vi "Main.vi"(8 "error in (no error)":errorcluster, 11 "TomoBase in":refnum<class "Tomo.lvclass">) -> (0 "error out":errorcluster, 3 "component":refnum<class "Tomo.lvclass">)   [LabVIEW 2012, in "Tomo.lvclass"]
doc: "Main VI of the component."
uses:
  Tomo.lvclass
  <vilib>/Distrio/Murmex/Murmex/command_enum.ctl
  Tomo.lvclass/Tomo.ctl
  <vilib>/Distrio/Murmex/InitialiseMessage/InitialiseMessage.lvclass
  <vilib>/Distrio/Murmex/TerminateMessage/TerminateMessage.lvclass
  <vilib>/Distrio/Murmex/ConfigureMessage/ConfigureMessage.lvclass
  <vilib>/Distrio/Murmex/Murmex/update_cluster.ctl
  <vilib>/Distrio/Murmex/StopMessage/StopMessage.lvclass
  <vilib>/Distrio/Murmex/GenericMessage/GenericMessage.lvclass
  <vilib>/Distrio/Murmex/Murmex/Set configure at initialise.vi
  <vilib>/Distrio/Murmex/Murmex/Set log reference.vi
  <vilib>/Distrio/Murmex/Murmex/Set VI reference.vi
  <vilib>/Distrio/Murmex/Message/Add or replace parameter.vi
  <vilib>/Distrio/Murmex/Murmex/Murmex.lvclass
  <vilib>/Distrio/Murmex/Message/Message.lvclass
panel:
  in  "Tab Control":T1(tab)
  out "TB":dbl format="%#_2g"
  out "Tomography progress":dbl(slide) scale=0.0..1.0
  in  "experiment name":string
  in  "Volume map":T2(ring)
  in  "Z step size":dbl[unit]=1e-06
  in  "X step size":dbl[unit]=0.0005
  in  "Y step size":dbl[unit]=0.0005
  in  "number of views":dbl=1.0
  in  "starting angle":dbl[unit]
  in  "button::start":bool
  out "Estimated remaining time":dbl format="- %<%H:%M:%S>t"
  in  "X min":dbl[unit]
  in  "X max":dbl[unit]
  in  "Y min":dbl[unit]
  in  "Y max":dbl[unit]
  in  "Z min":dbl[unit]
  in  "Z max":dbl[unit]
  in  "Custom volume path":path
  in  "generic command":string
  in  "button::send command":bool
  out "log":string
  in  "ID":string="tomo"
  in  "command":T3
  in  "recipient":string
  in  "button::configure":bool
  in  "button::quit":bool
  in  "terminate?":bool
  # "Tomo\n\nImplemented by:\nLudovico Silvestri\nUniversity of Florence, Italy"
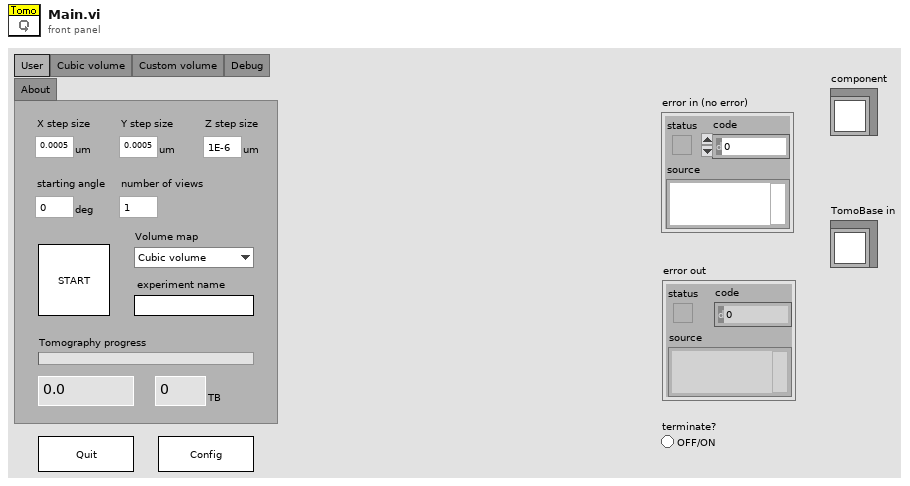
[diagram p1: front panel]
types:
  T1 = enum32{"User", "Cubic volume", "Custom volume", "Debug", "About"}
  T2 = enum16{"Cubic volume", "Custom volume", "Self-generate volume"}
  T3 = typedef "Murmex.lvlib/Murmex.lvclass/command_enum.ctl" = enum16{"null", "initialise", "reset", "terminate", "acknowledge", "update", "inspect", "inform", "proceed", "start", "stop", "fetch", "configure", "generic"}
  T4 = typedef "Murmex.lvlib/Murmex.lvclass/update_cluster.ctl" = cluster{"target ID":string, "key chains":string[], "values":variant[]}
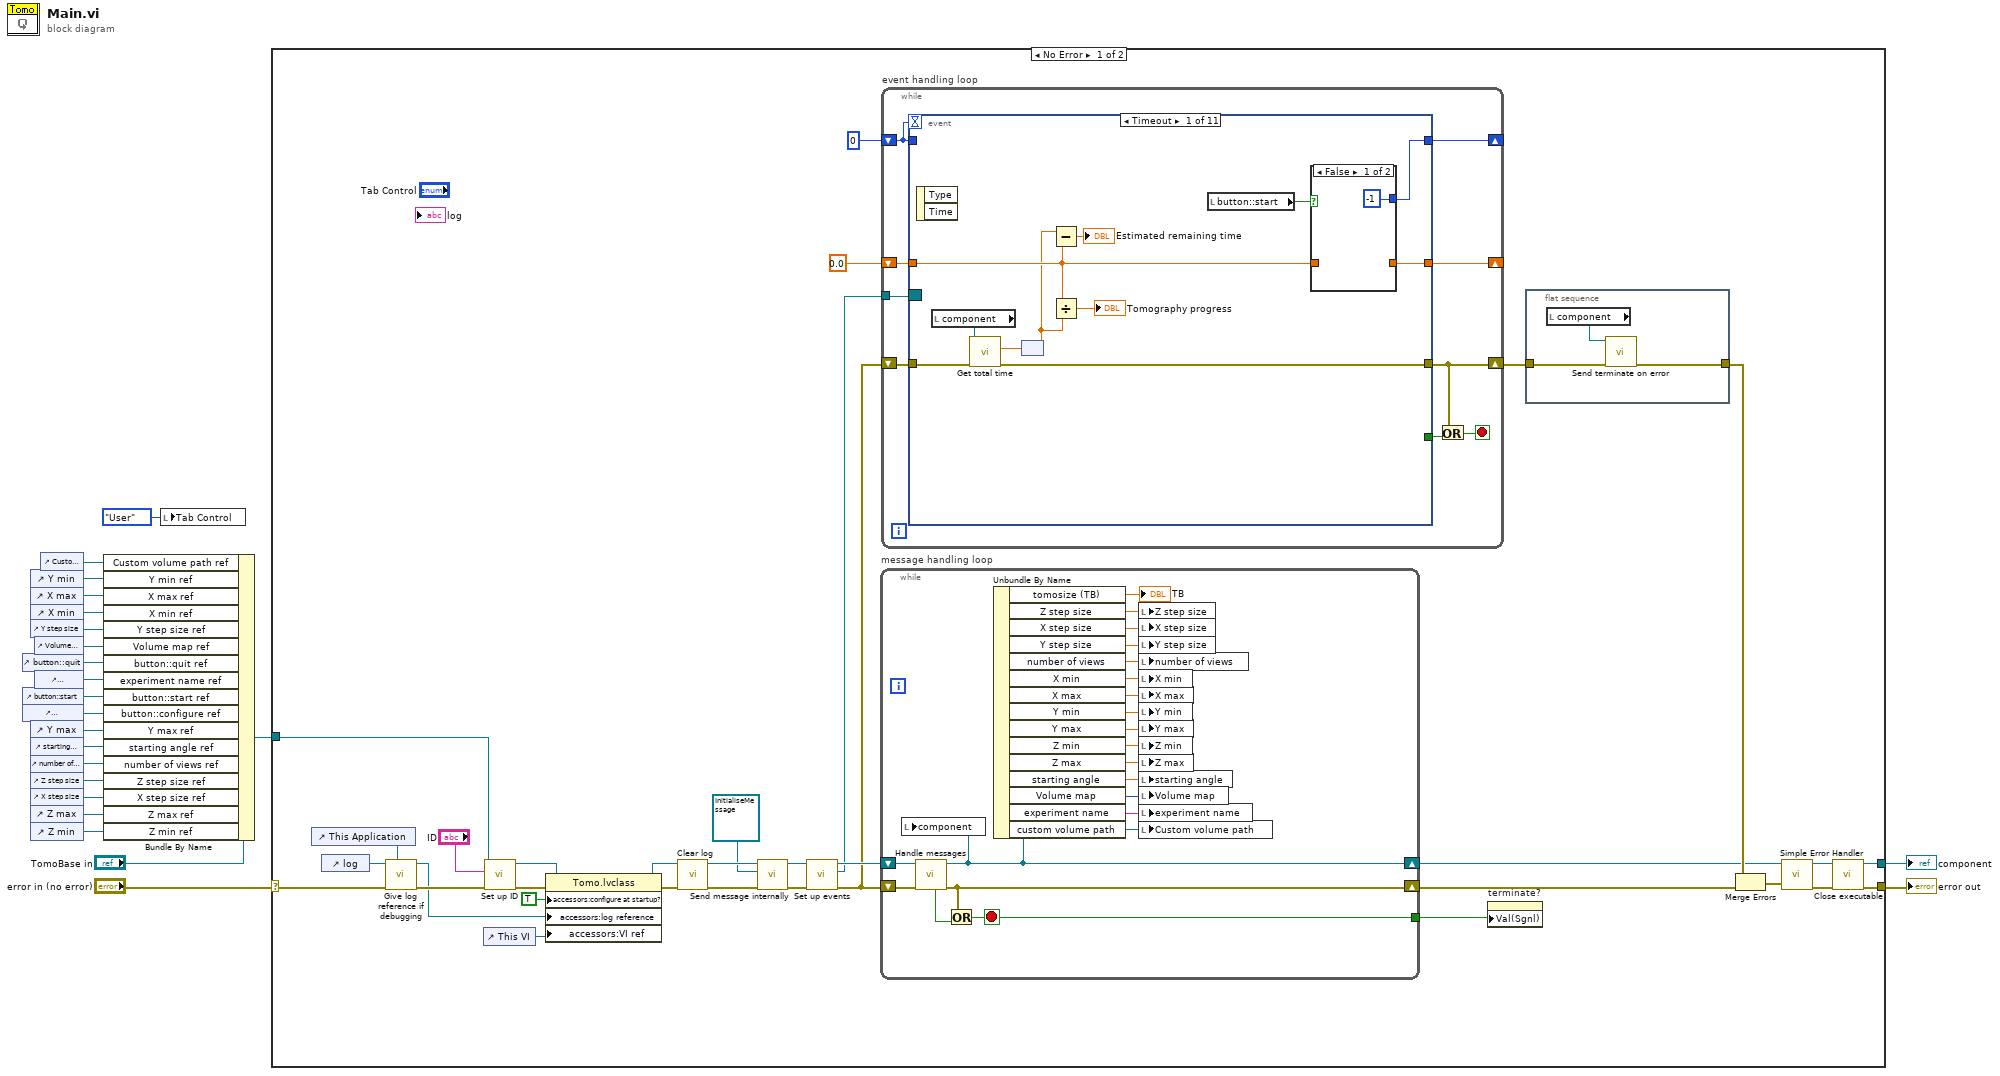
[diagram p0: block diagram]
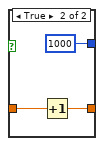
[diagram p2: hidden frame]
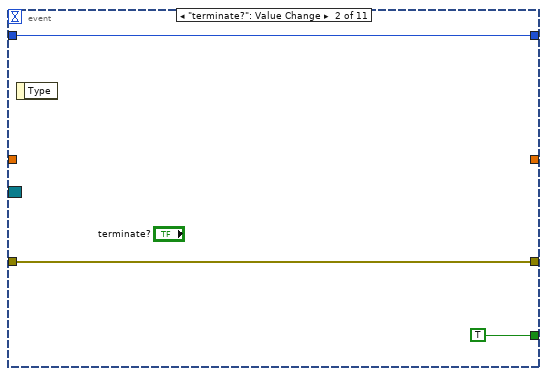
[diagram p3: hidden frame]
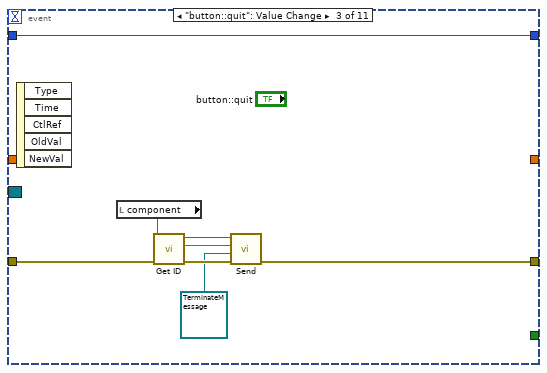
[diagram p4: hidden frame]
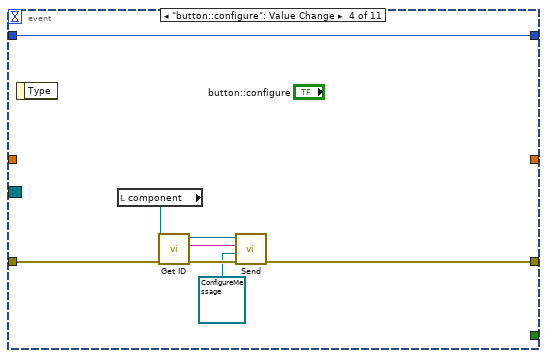
[diagram p5: hidden frame]
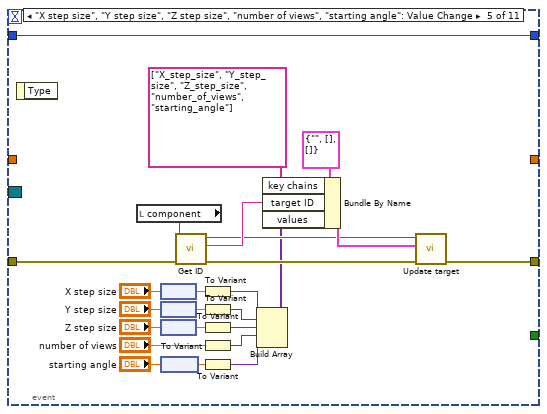
[diagram p6: hidden frame]
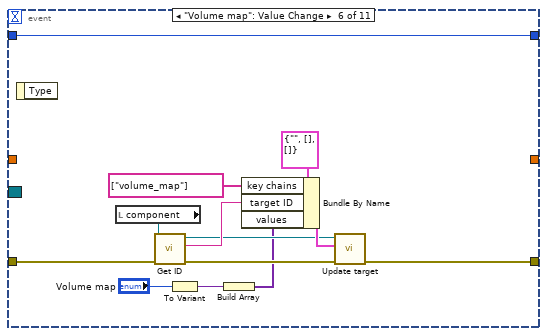
[diagram p7: hidden frame]
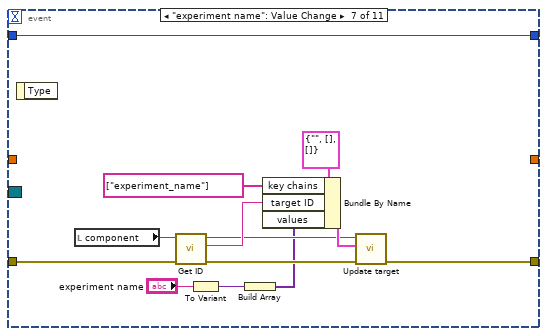
[diagram p8: hidden frame]
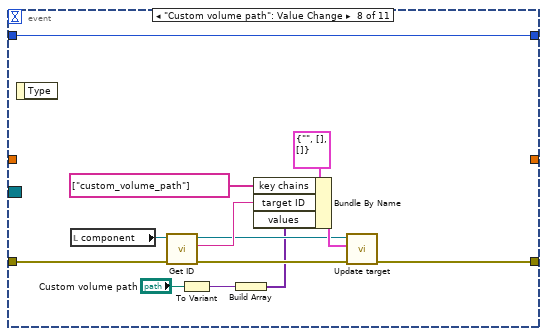
[diagram p9: hidden frame]
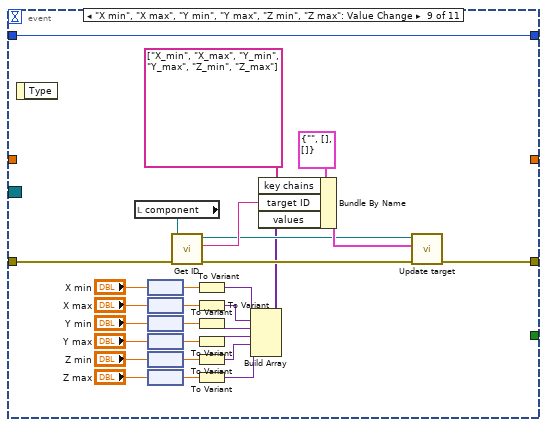
[diagram p10: hidden frame]
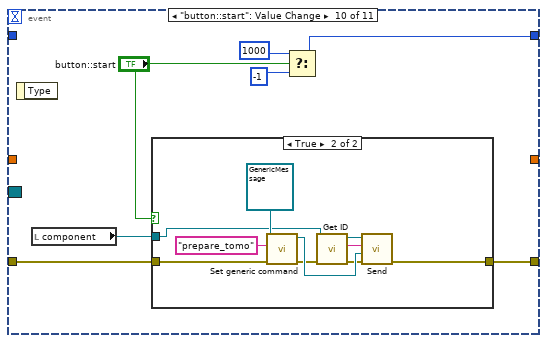
[diagram p11: hidden frame]
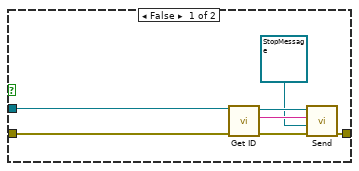
[diagram p12: hidden frame]
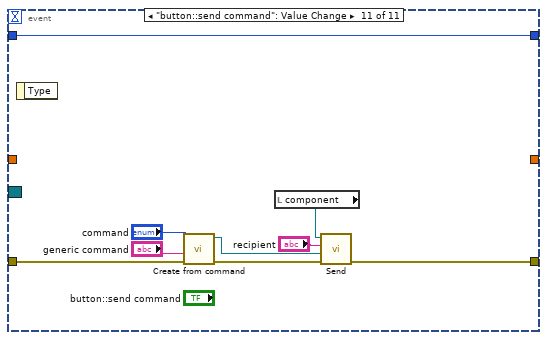
[diagram p13: hidden frame]
diagram:
  n1 = control-ref of="button::quit"() -> (w11:refnum<vi>)
  n2 = control-ref of="button::start"() -> (w9:refnum<vi>)
  n3 = control-ref of="button::configure"() -> (w8:refnum<vi>)
  n4 = control-ref of="Y min"() -> (w16:refnum<vi>)
  n5 = control-ref of="X max"() -> (w15:refnum<vi>)
  n6 = control-ref of="X min"() -> (w14:refnum<vi>)
  n7 = control-ref of="Y step size"() -> (w13:refnum<vi>)
  n8 = control-ref of="Y max"() -> (w7:refnum<vi>)
  n9 = control-ref of="starting angle"() -> (w6:refnum<vi>)
  n10 = control-ref of="number of views"() -> (w5:refnum<vi>)
  n11 = control-ref of="Z step size"() -> (w4:refnum<vi>)
  n12 = control-ref of="X step size"() -> (w3:refnum<vi>)
  n13 = control-ref of="Z max"() -> (w2:refnum<vi>)
  n14 = control-ref of="Z min"() -> (w1:refnum<vi>)
  n15 = control-ref of="Volume map"() -> (w12:refnum<vi>)
  n16 = control-ref of="experiment name"() -> (w10:refnum<vi>)
  n17 = control-ref of="Custom volume path"() -> (w17:refnum<vi>)
  n18 = Bundle By Name(cluster="TomoBase in", "Custom volume path ref"=w17, "Y min ref"=w16, "X max ref"=w15, "X min ref"=w14, "Y step size ref"=w13, "Volume map ref"=w12, "button::quit ref"=w11, "experiment name ref"=w10, "button::start ref"=w9, "button::configure ref"=w8, "Y max ref"=w7, "starting angle ref"=w6, "number of views ref"=w5, "Z step size ref"=w4, "X step size ref"=w3, "Z max ref"=w2, "Z min ref"=w1) -> (w18:refnum<class "Tomo.lvclass">)
  n19 = local write "Tab Control"(T1."User" ("Tab Control")) -> ()
  n20 = case shown="No Error" "error in (no error)" {
    selector: "error in (no error)" -> [w27 w250]
    tunnel: w18 -> [w52 w249]
    tunnel: [w32 w250] -> w22
    tunnel: [w30 w249] -> w21
    frame No Error {
      n21 = control-ref of="This Application"() -> (w24:refnum<vi>)
      n22 = control-ref of="log"() -> (w26:refnum<vi>)
      n23 = call "Give log reference if debugging.vi"("application ref"=w24, "error in (no error)"=w27, "log reference in"=w26) -> ("error out"=w28:errorcluster, "log reference out"=w25:refnum<vi>)  [unwired: 6 in, 1 out]
      n24 = control-ref of="This VI"() -> (w54:refnum<vi>)
      n25 = call <vilib>:"Set up ID.vi"("error in (no error)"=w28, "component ID"="ID", "MurmexBase in"=w52) -> ("error out"=w53:errorcluster, "MurmexBase out"=w50:refnum<class "Tomo.lvclass">)  [unwired: 6 in, 1 out]
      n26 = property class="Tomo.lvclass"(reference=w50, error in=w53, "accessors:configure at startup?"=TRUE ("configure at startup?"), "accessors:log reference"=w25, "accessors:VI ref"=w54) -> (reference out=w48:refnum<class "Tomo.lvclass">, error out=w49:errorcluster)
      n27 = call <vilib>:"Clear log.vi"("error in (no error)"=w49, "MurmexBase in"=w48) -> ("error out"=w47:errorcluster, "MurmexBase out"=w46:refnum<class "Tomo.lvclass">)  [unwired: 8 in]
      n28 = call <vilib>:"Send message internally.vi"("error in (no error)"=w47, "Message"=refnum<class "InitialiseMessage.lvclass"> refnum ("Message in"), "Murmex in"=w46) -> ("error out"=w44:errorcluster, "Murmex out"=w43:refnum<class "Tomo.lvclass">)  [unwired: 7 in]
      n29 = call <vilib>:"Set up events.vi"("error in (no error)"=w44, "MurmexBase in"=w43) -> ("error out"=w41:errorcluster, "Event Registration Refnum"=w40:refnum<event-registration>, "MurmexBase out"=w42:refnum<class "Tomo.lvclass">)  [unwired: 7 in]
      n30 = while "message handling loop" {
        shift-right: [w245] -> w37
        shift-left: w41 -> [w248]
        shift-right: [w243] -> w31
        shift-left: w42 -> [w247]
        tunnel: [w244] -> w33
        stop <- w244 stop-if-true
        n31 = call <vilib>:"Handle messages.vi"("error in (no error)"=w248, "Murmex in"=w247) -> ("error out"=w245:errorcluster, "Murmex out"=w243:refnum<class "Tomo.lvclass">, "terminated?"=w246:bool)  [unwired: 7 in]
        n32 = local write "component"(w243) -> ()
        n33 = Or(x=w245, y=w246) -> (x .or. y?=w244:bool)
        n34 = Unbundle By Name(w243) -> ("tomosize (TB)"=→"TB":dbl, "Z step size"=w234:dbl[unit], "X step size"=w236:dbl[unit], "Y step size"=w235:dbl[unit], "number of views"=w233:dbl, "X min"=w242:dbl[unit], "X max"=w241:dbl[unit], "Y min"=w240:dbl[unit], "Y max"=w239:dbl[unit], "Z min"=w238:dbl[unit], "Z max"=w237:dbl[unit], "starting angle"=w232:dbl[unit], "Volume map"=w231:T2, "experiment name"=w230:string, "custom volume path"=w229:path)
        n35 = local write "Z step size"(w234) -> ()
        n36 = local write "X step size"(w236) -> ()
        n37 = local write "Y step size"(w235) -> ()
        n38 = local write "number of views"(w233) -> ()
        n39 = local write "X min"(w242) -> ()
        n40 = local write "X max"(w241) -> ()
        n41 = local write "Y min"(w240) -> ()
        n42 = local write "Y max"(w239) -> ()
        n43 = local write "Z min"(w238) -> ()
        n44 = local write "Z max"(w237) -> ()
        n45 = local write "starting angle"(w232) -> ()
        n46 = local write "Volume map"(w231) -> ()
        n47 = local write "experiment name"(w230) -> ()
        n48 = local write "Custom volume path"(w229) -> ()
      }
      n49 = while "event handling loop" {
        shift-right: [w62] -> w38
        shift-left: w41 -> [w67]
        tunnel: w40 -> [w66]
        shift-right: [w64] -> _
        shift-left: 0 -> [w65]
        shift-right: [w59] -> _
        shift-left: 0.0 -> [w60]
        stop <- w61 stop-if-true
        n50 = event shown="[0] Timeout" {
          selector: w66 -> [_ _ _ _ _ _ _ _ _ _ _]
          dyn-events: _ -> [_ _ _ _ _ _ _ _ _ _ _]
          timeout: w65 -> [_ _ _ _ _ _ _ _ _ _ _]
          tunnel: [w77 w84 w91 w97 w125 w134 w142 w158 w189 w201 w220] -> w62
          tunnel: w67 -> [w78 w84 w93 w98 w123 w136 w145 w157 w187 w200 w226]
          tunnel: w65 -> [_ w83 w86 w94 w106 w133 w141 w153 w173 _ w219]
          tunnel: [w76 w83 w86 w94 w106 w133 w141 w153 w173 w195 w219] -> w64
          tunnel: [_ TRUE _ _ _ _ _ _ _ _ _] -> w63
          tunnel: w60 -> [w75 _ _ _ _ _ _ _ _ _ _]
          tunnel: [w74 _ _ _ _ _ _ _ _ _ _] -> w59
          event Timeout {
            n51 = event-data() -> ()  [unwired: 1 in, 2 out]
            n52 = local read "component"() -> (w73:refnum<class "Tomo.lvclass">)
            n53 = call-dynamic "Get total time.vi"("error in (no error)"=w78, "Tomo in"=w73) -> ("error out"=w77:errorcluster, "Total time"=w72:dbl[unit])  [unwired: 7 in, 1 out]
            n54 = node(w72) -> (w70:dbl)
            n55 = Subtract(x=w70, y=w75) -> (x-y=→"Estimated remaining time":dbl)
            n56 = Divide(x=w75, y=w70) -> (x/y=→"Tomography progress":dbl)
            n57 = local read "button::start"() -> (w68:bool)
            n58 = case shown="False" w68 {
              tunnel: [-1 1000] -> w76
              tunnel: w75 -> [_ w81]
              tunnel: [_ w80] -> w74
              frame False {
              }
              frame True {
                n59 = Increment(x=w81) -> (x+1=w80:dbl)
              }
            }
          }
          event "terminate?": Value Change {
            n60 = event-data() -> ()  [unwired: 1 in, 1 out]
          }
          event "button::quit": Value Change {
            n61 = event-data() -> ()  [unwired: 1 in, 5 out]
            n62 = local read "component"() -> (w90:refnum<class "Tomo.lvclass">)
            n63 = call <vilib>:"Get ID.vi"("error in (no error)"=w93, "Murmex in"=w90) -> ("error out"=w92:errorcluster, "component id"=w88:string, "Murmex out"=w89:refnum<class "Tomo.lvclass">)  [unwired: 7 in]
            n64 = call <vilib>:"Send.vi"("error in (no error)"=w92, "Message"=refnum<class "TerminateMessage.lvclass"> refnum ("Distrio Murmex 1.1:TerminateMessage"), "recipient"=w88, "Murmex in"=w89) -> ("error out"=w91:errorcluster)  [unwired: 6 in, 1 out]
          }
          event "button::configure": Value Change {
            n65 = event-data() -> ()  [unwired: 1 in, 1 out]
            n66 = local read "component"() -> (w96:refnum<class "Tomo.lvclass">)
            n67 = call <vilib>:"Get ID.vi"("error in (no error)"=w98, "Murmex in"=w96) -> ("error out"=w101:errorcluster, "component id"=w99:string, "Murmex out"=w100:refnum<class "Tomo.lvclass">)  [unwired: 7 in]
            n68 = call <vilib>:"Send.vi"("error in (no error)"=w101, "Message"=refnum<class "ConfigureMessage.lvclass"> refnum ("Distrio Murmex 1.1:ConfigureMessage"), "recipient"=w99, "Murmex in"=w100) -> ("error out"=w97:errorcluster)  [unwired: 6 in, 1 out]
          }
          event "X step size", "Y step size", "Z step size", "number of views", "starting angle": Value Change {
            n69 = event-data() -> ()  [unwired: 1 in, 1 out]
            n70 = local read "component"() -> (w121:refnum<class "Tomo.lvclass">)
            n71 = node("X step size") -> (w105:dbl)
            n72 = node("Y step size") -> (w104:dbl)
            n73 = node("Z step size") -> (w103:dbl)
            n74 = node("starting angle") -> (w102:dbl)
            n75 = call <vilib>:"Get ID.vi"("error in (no error)"=w123, "Murmex in"=w121) -> ("error out"=w124:errorcluster, "component id"=w122:string, "Murmex out"=w119:refnum<class "Tomo.lvclass">)  [unwired: 7 in]
            n76 = To Variant(anything=w105) -> (Variant=w109:variant)
            n77 = To Variant(anything=w104) -> (Variant=w110:variant)
            n78 = To Variant(anything=w103) -> (Variant=w113:variant)
            n79 = To Variant(anything="number of views") -> (Variant=w112:variant)
            n80 = To Variant(anything=w102) -> (Variant=w111:variant)
            n81 = Build Array(w109, w110, w113, w112, w111) -> (w108:variant[])
            n82 = Bundle By Name(cluster=T4 {"target ID"="", "key chains"=[], "values"=[]} ("update cluster"), "key chains"=string[] ["X_step_size", "Y_step_size", "Z_step_size", "number_of_views", "starting_angle"], "target ID"=w122, "values"=w108) -> (w120:T4)
            n83 = call <vilib>:"Update target.vi"("error in (no error)"=w124, "update cluster"=w120, "MurmexBase in"=w119) -> ("error out"=w125:errorcluster)  [unwired: 7 in, 1 out]
          }
          event "Volume map": Value Change {
            n84 = event-data() -> ()  [unwired: 1 in, 1 out]
            n85 = local read "component"() -> (w127:refnum<class "Tomo.lvclass">)
            n86 = call <vilib>:"Get ID.vi"("error in (no error)"=w136, "Murmex in"=w127) -> ("error out"=w135:errorcluster, "component id"=w139:string, "Murmex out"=w137:refnum<class "Tomo.lvclass">)  [unwired: 7 in]
            n87 = To Variant(anything="Volume map") -> (Variant=w132:variant)
            n88 = Build Array(w132) -> (w131:variant[])
            n89 = Bundle By Name(cluster=T4 {"target ID"="", "key chains"=[], "values"=[]} ("update cluster"), "key chains"=string[] ["volume_map"], "target ID"=w139, "values"=w131) -> (w138:T4)
            n90 = call <vilib>:"Update target.vi"("error in (no error)"=w135, "update cluster"=w138, "MurmexBase in"=w137) -> ("error out"=w134:errorcluster)  [unwired: 7 in, 1 out]
          }
          event "experiment name": Value Change {
            n91 = event-data() -> ()  [unwired: 1 in, 1 out]
            n92 = local read "component"() -> (w140:refnum<class "Tomo.lvclass">)
            n93 = call <vilib>:"Get ID.vi"("error in (no error)"=w145, "Murmex in"=w140) -> ("error out"=w149:errorcluster, "component id"=w152:string, "Murmex out"=w150:refnum<class "Tomo.lvclass">)  [unwired: 7 in]
            n94 = To Variant(anything="experiment name") -> (Variant=w148:variant)
            n95 = Build Array(w148) -> (w147:variant[])
            n96 = Bundle By Name(cluster=T4 {"target ID"="", "key chains"=[], "values"=[]} ("update cluster"), "key chains"=string[] ["experiment_name"], "target ID"=w152, "values"=w147) -> (w151:T4)
            n97 = call <vilib>:"Update target.vi"("error in (no error)"=w149, "update cluster"=w151, "MurmexBase in"=w150) -> ("error out"=w142:errorcluster)  [unwired: 7 in, 1 out]
          }
          event "Custom volume path": Value Change {
            n98 = event-data() -> ()  [unwired: 1 in, 1 out]
            n99 = local read "component"() -> (w155:refnum<class "Tomo.lvclass">)
            n100 = call <vilib>:"Get ID.vi"("error in (no error)"=w157, "Murmex in"=w155) -> ("error out"=w162:errorcluster, "component id"=w165:string, "Murmex out"=w163:refnum<class "Tomo.lvclass">)  [unwired: 7 in]
            n101 = To Variant(anything="Custom volume path") -> (Variant=w161:variant)
            n102 = Build Array(w161) -> (w160:variant[])
            n103 = Bundle By Name(cluster=T4 {"target ID"="", "key chains"=[], "values"=[]} ("update cluster"), "key chains"=string[] ["custom_volume_path"], "target ID"=w165, "values"=w160) -> (w164:T4)
            n104 = call <vilib>:"Update target.vi"("error in (no error)"=w162, "update cluster"=w164, "MurmexBase in"=w163) -> ("error out"=w158:errorcluster)  [unwired: 7 in, 1 out]
          }
          event "X min", "X max", "Y min", "Y max", "Z min", "Z max": Value Change {
            n105 = event-data() -> ()  [unwired: 1 in, 1 out]
            n106 = local read "component"() -> (w186:refnum<class "Tomo.lvclass">)
            n107 = node("X min") -> (w172:dbl)
            n108 = node("X max") -> (w171:dbl)
            n109 = node("Y min") -> (w170:dbl)
            n110 = node("Y max") -> (w169:dbl)
            n111 = node("Z min") -> (w167:dbl)
            n112 = node("Z max") -> (w166:dbl)
            n113 = call <vilib>:"Get ID.vi"("error in (no error)"=w187, "Murmex in"=w186) -> ("error out"=w188:errorcluster, "component id"=w193:string, "Murmex out"=w191:refnum<class "Tomo.lvclass">)  [unwired: 7 in]
            n114 = To Variant(anything=w172) -> (Variant=w182:variant)
            n115 = To Variant(anything=w171) -> (Variant=w183:variant)
            n116 = To Variant(anything=w170) -> (Variant=w185:variant)
            n117 = To Variant(anything=w169) -> (Variant=w184:variant)
            n118 = To Variant(anything=w167) -> (Variant=w175:variant)
            n119 = To Variant(anything=w166) -> (Variant=w174:variant)
            n120 = Build Array(w182, w183, w185, w184, w175, w174) -> (w181:variant[])
            n121 = Bundle By Name(cluster=T4 {"target ID"="", "key chains"=[], "values"=[]} ("update cluster"), "key chains"=string[] ["X_min", "X_max", "Y_min", "Y_max", "Z_min", "Z_max"], "target ID"=w193, "values"=w181) -> (w192:T4)
            n122 = call <vilib>:"Update target.vi"("error in (no error)"=w188, "update cluster"=w192, "MurmexBase in"=w191) -> ("error out"=w189:errorcluster)  [unwired: 7 in, 1 out]
          }
          event "button::start": Value Change {
            n123 = event-data() -> ()  [unwired: 1 in, 1 out]
            n124 = local read "component"() -> (w199:refnum<class "Tomo.lvclass">)
            n125 = case shown="True" "button::start" {
              tunnel: [w206 w209] -> w201
              tunnel: w200 -> [w204 w211]
              tunnel: w199 -> [w202 w210]
              frame False {
                n126 = call <vilib>:"Get ID.vi"("error in (no error)"=w204, "Murmex in"=w202) -> ("error out"=w205:errorcluster, "component id"=w207:string, "Murmex out"=w208:refnum<class "Tomo.lvclass">)  [unwired: 7 in]
                n127 = call <vilib>:"Send.vi"("error in (no error)"=w205, "Message"=refnum<class "StopMessage.lvclass"> refnum ("Distrio Murmex 1.1:StopMessage"), "recipient"=w207, "Murmex in"=w208) -> ("error out"=w206:errorcluster)  [unwired: 6 in, 1 out]
              }
              frame True {
                n128 = call <vilib>:"Set generic command.vi"("error in (no error)"=w211, "generic command"="prepare_tomo", "GenericMessage in"=refnum<class "GenericMessage.lvclass"> refnum ("Message in")) -> ("error out"=w213:errorcluster, "GenericMessage out"=w217:refnum<class "GenericMessage.lvclass">)  [unwired: 7 in]
                n129 = call <vilib>:"Get ID.vi"("error in (no error)"=w213, "Murmex in"=w210) -> ("error out"=w214:errorcluster, "component id"=w216:string, "Murmex out"=w215:refnum<class "Tomo.lvclass">)  [unwired: 7 in]
                n130 = call <vilib>:"Send.vi"("error in (no error)"=w214, "Message"=w217, "recipient"=w216, "Murmex in"=w215) -> ("error out"=w209:errorcluster)  [unwired: 6 in, 1 out]
              }
            }
            n131 = Select(t=1000, s="button::start", f=-1) -> (s? t:f=w195:i32)
          }
          event "button::send command": Value Change {
            n132 = event-data() -> ()  [unwired: 1 in, 1 out]
            n133 = call <vilib>:"Create from command.vi"("error in (no error)"=w226, "generic command"="generic command", "command"="command") -> ("error out"=w221:errorcluster, "Message out"=w222:refnum<class "Message.lvclass">)  [unwired: 7 in]
            n134 = local read "component"() -> (w223:refnum<class "Tomo.lvclass">)
            n135 = call <vilib>:"Send.vi"("error in (no error)"=w221, "Message"=w222, "recipient"="recipient", "Murmex in"=w223) -> ("error out"=w220:errorcluster)  [unwired: 6 in, 1 out]
          }
        }
        n136 = Or(x=w62, y=w63) -> (x .or. y?=w61:bool)
      }
      n137 = property on="terminate?" class="Bool (strict)"("Val(Sgnl)"=w33) -> ()  [unwired: 2 in, 2 out]
      n138 = flat-sequence {
        tunnel: w38 -> [w58]
        tunnel: [w56] -> w36
        frame #0 {
          n139 = local read "component"() -> (w57:refnum<class "Tomo.lvclass">)
          n140 = call <vilib>:"Send terminate on error.vi"("error in (no error)"=w58, "Murmex in"=w57) -> ("error out"=w56:errorcluster)  [unwired: 8 in, 1 out]
        }
      }
      n141 = Merge Errors(w36, w37) -> (w35:errorcluster)
      n142 = call <vilib>:"Simple Error Handler.vi"("error in (no error)"=w35) -> ("error out"=w34:errorcluster)  [unwired: 4 in, 4 out]
      n143 = call <vilib>:"Close executable.vi"("error in (no error)"=w34, "MurmexBase in"=w31) -> ("error out"=w32:errorcluster, "MurmexBase out"=w30:refnum<class "Tomo.lvclass">)  [unwired: 8 in]
    }
    frame Error {
    }
  }
  "error out" <- w22
  "component" <- w21
